vi "condition.vi"() -> ()   [LabVIEW 2022 SP3]
panel:
  out "数组 4":i32[](array[numeric])
  out "数组 3":i32[](array[numeric])
  out "数组 2":i32[][](array[numeric])
  out "数组":i32[](array[numeric])
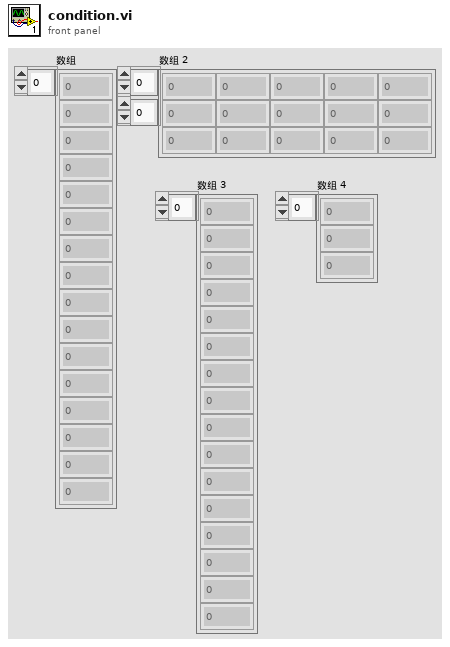
[diagram p1: front panel]
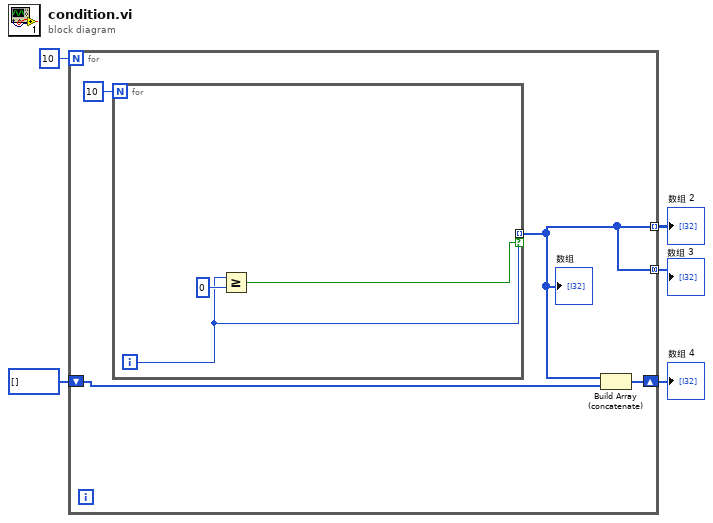
[diagram p0: block diagram]
diagram:
  n1 = for {
    N: 10 -> [_]
    tunnel: [w8] -> w4 mode=indexing
    tunnel: [w8] -> w3 mode=concatenating
    shift-right: [w7] -> w1
    shift-left: i32[] [] -> [w6]
    n2 = for {
      N: 10 -> [_]
      tunnel: [w11] -> w8 mode=indexing if=w10
      i -> [w11]
      n3 = Greater Or Equal?(x=w11, y=0) -> (x >= y?=w10:bool)
    }
    "数组" <- w8
    n4 = Build Array (concatenate)(w8, w6) -> (w7:i32[])
  }
  "数组 2" <- w4
  "数组 3" <- w3
  "数组 4" <- w1
